vi "Read Enclosure Door.vi"(4 "error in":errorcluster) -> (0 "error out":errorcluster, 2 "Enclosure Door Shut?":bool)   [LabVIEW 2015]
uses:
  <vilib>/DAQmx/read.llb/DAQmx Read (Digital Bool 1Line 1Point).vi
  <vilib>/DAQmx/miscellaneous.llb/DAQmx Fill In Error Info.vi
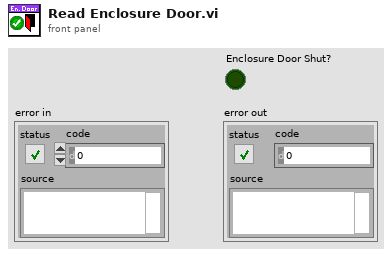
[diagram p1: front panel]
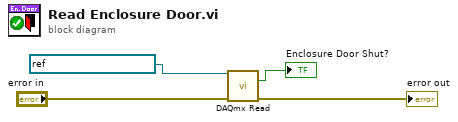
[diagram p0: block diagram]
diagram:
  n1 = call-poly <vilib>:"DAQmx Read.vi"("task/channels in"=refnum<k21> "DI6 Enclosure Shut" ("DAQmx Global Channel"), "error in"="error in") -> ("data"=→"Enclosure Door Shut?":bool, "error out"=→"error out":errorcluster)  [unwired: 11 in, 1 out]
